vi "Connection Loop Async.vi"(11 "TCP Client in":refnum<class "TCP Client.lvclass">) -> ()   [LabVIEW 2020, in "Stream-TCP.lvlib" / "TCP Client.lvclass"]
uses:
  TCP Client.lvclass
  C:/dev/LabVIEW/lv-stream/stream/Endpoint/Endpoint.lvclass
  C:/dev/LabVIEW/lv-stream/stream/Connection/Connection.lvclass
  Connection State.ctl
  lv-stream/stream/Connection State.ctl
  TCP Client.lvclass/TCP Client.ctl
  lv-stream/stream/Endpoint/Endpoint.lvclass
  lv-stream/stream/URI/URI.lvclass
  TCP Stream/TCP Stream.lvclass
  lv-stream/stream/Connection/Connection.lvclass
  lv-stream/stream/Stream.lvlib
panel:
  out "URI String":string
  out "State":T1
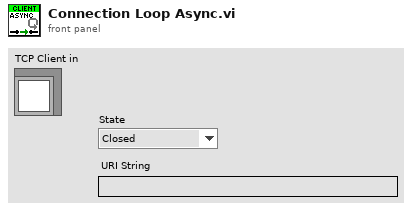
[diagram p1: front panel]
types:
  T1 = typedef "Stream-TCP.lvlib/TCP Client.lvclass/Connection State.ctl" = enum16{"Closed", "Idle", "Connecting", "Connected", "Shutdown"}
  T2 = typedef "Stream.lvlib/Connection State.ctl" = enum16{"Connected", "Disconnected"}
  T3 = typedef "Stream-TCP.lvlib/Client Command.ctl" = enum16{"Connect", "Close", "Shutdown", "Reconnect"}
  T4 = typedef "Stream-TCP.lvlib/Client Command Queue.ctl" = refnum<queue>
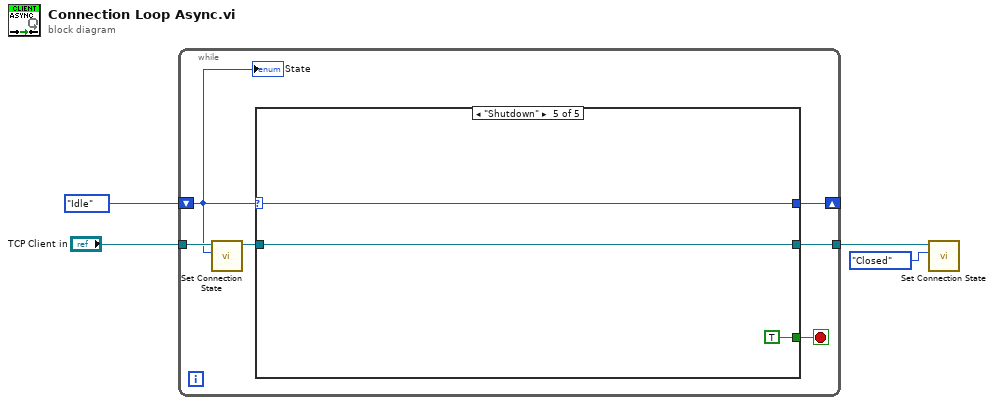
[diagram p0: block diagram]
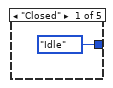
[diagram p2: hidden frame]
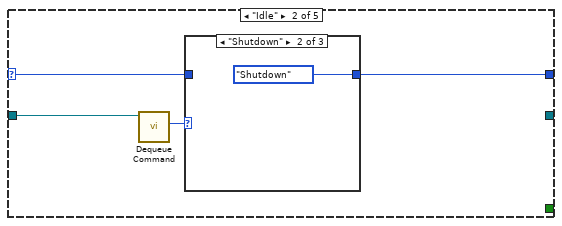
[diagram p3: hidden frame]
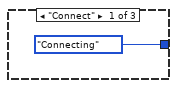
[diagram p4: hidden frame]
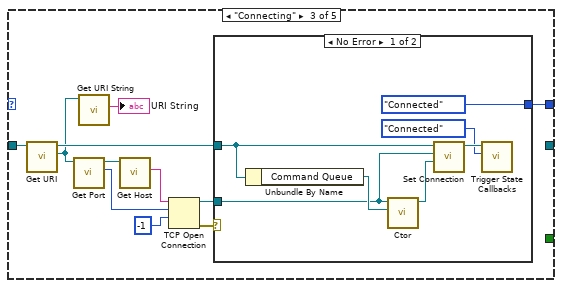
[diagram p6: hidden frame]
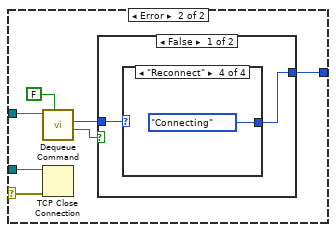
[diagram p7: hidden frame]
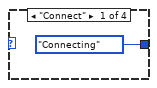
[diagram p8: hidden frame]
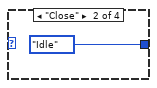
[diagram p9: hidden frame]
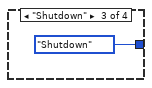
[diagram p10: hidden frame]
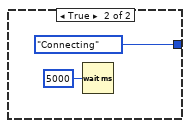
[diagram p11: hidden frame]
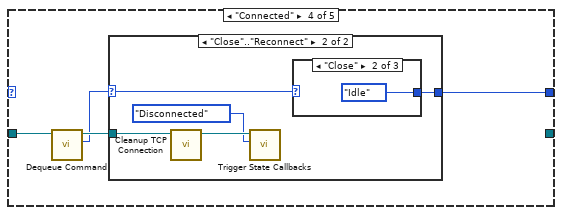
[diagram p12: hidden frame]
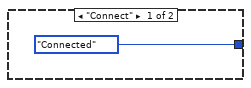
[diagram p13: hidden frame]
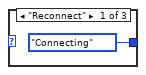
[diagram p14: hidden frame]
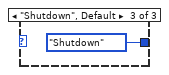
[diagram p15: hidden frame]
diagram:
  n1 = while {
    tunnel: "TCP Client in" -> [w8]
    shift-right: [w5] -> _
    shift-left: Connection_State."Idle" ("Connection State") -> [w6]
    tunnel: [w9] -> w3
    stop <- w10 stop-if-true
    n2 = call "Set Connection State.vi"("Connection State"=w6, "TCP Client in"=w8) -> ("TCP Client out"=w7:refnum<class "TCP Client.lvclass">)  [unwired: 8 in, 1 out]
    n3 = case shown="\"Shutdown\"" w6 {
      selector: w6 -> [_ w13 _ _ w65]
      tunnel: [_ _ _ _ TRUE] -> w10
      tunnel: w7 -> [_ w15 w28 w54 w66]
      tunnel: [_ _ _ _ w66] -> w9
      tunnel: [Connection_State."Idle" ("Connection State") w12 w21 w55 w65] -> w5
      frame "Closed" {
      }
      frame "Idle" {
        n4 = call "Dequeue Command.vi"("TCP Client in"=w15) -> ("Command"=w14:T3)  [unwired: 7 in, 3 out]
        n5 = case shown="\"Shutdown\"" w14 {
          tunnel: [Connection_State."Connecting" ("Connection State") Connection_State."Shutdown" ("Connection State") w18] -> w12
          tunnel: w13 -> [_ _ w18]
          frame "Connect" {
          }
          frame "Shutdown" {
          }
          frame Default {
          }
        }
      }
      frame "Connecting" {
        n6 = call "Get URI.vi"("Endpoint in"=w28) -> ("URI"=w20:refnum<class "URI.lvclass">, "Endpoint out"=w23:refnum<class "TCP Client.lvclass">)  [unwired: 8 in, 1 out]
        n7 = call "Get Port.vi"("URI in"=w20) -> ("Port"=w25:u16, "URI out"=w27:refnum<class "URI.lvclass">)  [unwired: 8 in, 1 out]
        n8 = call "Get URI String.vi"("URI in"=w20) -> ("URI String"=→"URI String":string)  [unwired: 8 in, 2 out]
        n9 = call "Get Host.vi"("URI in"=w27) -> ("Host"=w26:string)  [unwired: 8 in, 2 out]
        n10 = TCP Open Connection(address=w26, remote port or service name=w25, timeout ms (60000)=-1) -> (connection ID=w22:refnum<k5>, error out=w24:errorcluster)  [unwired: 2 in]
        n11 = case shown="No Error" w24 {
          selector: w24 -> [_ w37]
          tunnel: w23 -> [w34 w42]
          tunnel: w22 -> [w32 w38]
          tunnel: [Connection_State."Connected" ("Connection State") w43] -> w21
          frame No Error {
            n12 = Unbundle By Name(w34) -> ("Command Queue"=w36:T4)
            n13 = call "Ctor.vi"("Client Command Queue"=w36, "TCP Connection"=w32) -> ("TCP Stream out"=w33:refnum<class "TCP Stream.lvclass">)  [unwired: 8 in, 1 out]
            n14 = call "Set Connection.vi"("TCP Stream"=w33, "TCP Connection"=w32, "TCP Client in"=w34) -> ("TCP Client out"=w31:refnum<class "TCP Client.lvclass">)  [unwired: 7 in, 1 out]
            n15 = call "Trigger State Callbacks.vi"("State"=Connection_State."Connected", "Connection in"=w31) -> ()  [unwired: 8 in, 2 out]
          }
          frame Error {
            n16 = call "Dequeue Command.vi"("Wait? (T)"=FALSE, "TCP Client in"=w42) -> ("timed out?"=w40:bool, "Command"=w39:T3)  [unwired: 6 in, 2 out]
            n17 = TCP Close Connection(connection ID=w38, error in (no error)=w37) -> ()  [unwired: 1 in, 2 out]
            n18 = case shown="False" w40 {
              tunnel: [w44 Connection_State."Connecting" ("Connection State")] -> w43
              tunnel: w39 -> [w45 _]
              frame False {
                n19 = case shown="\"Reconnect\"" w45 {
                  tunnel: [Connection_State."Connecting" ("Connection State") Connection_State."Idle" ("Connection State") Connection_State."Shutdown" ("Connection State") Connection_State."Connecting" ("Connection State")] -> w44
                  frame "Connect" {
                  }
                  frame "Close" {
                  }
                  frame "Shutdown" {
                  }
                  frame "Reconnect" {
                  }
                }
              }
              frame True {
                n20 = Wait (ms)(milliseconds to wait=u32 5000) -> ()  [unwired: 1 out]
              }
            }
          }
        }
      }
      frame "Connected" {
        n21 = call "Dequeue Command.vi"("TCP Client in"=w54) -> ("Command"=w52:T3, "TCP Client out"=w53:refnum<class "TCP Client.lvclass">)  [unwired: 7 in, 2 out]
        n22 = case shown="\"Close\"..\"Reconnect\"" w52 {
          selector: w52 -> [_ w57]
          tunnel: [Connection_State."Connected" ("Connection State") w61] -> w55
          tunnel: w53 -> [_ w58]
          frame "Connect" {
          }
          frame "Close".."Reconnect" {
            n23 = call "Cleanup TCP Connection.vi"("TCP Client in"=w58) -> ("TCP Client out"=w60:refnum<class "TCP Client.lvclass">)  [unwired: 9 in, 1 out]
            n24 = call "Trigger State Callbacks.vi"("State"=Connection_State."Disconnected", "Connection in"=w60) -> ()  [unwired: 8 in, 2 out]
            n25 = case shown="\"Close\"" w57 {
              tunnel: [Connection_State."Connecting" ("Connection State") Connection_State."Idle" ("Connection State") Connection_State."Shutdown" ("Connection State")] -> w61
              frame "Reconnect" {
              }
              frame "Close" {
              }
              frame "Shutdown", Default {
              }
            }
          }
        }
      }
      frame "Shutdown" {
      }
    }
    "State" <- w6
  }
  n26 = call "Set Connection State.vi"("Connection State"=Connection_State."Closed", "TCP Client in"=w3) -> ()  [unwired: 8 in, 2 out]
